vi "Set Variant.vi"(8 "error in (no error)":errorcluster, 10 "Variant":variant, 11 "int32 in":refnum<class "int32.lvclass">) -> (0 "error out":errorcluster, 3 "int32 out":refnum<class "int32.lvclass">)   [LabVIEW 2020, in "Protobuf RAW.lvlib" / "int32.lvclass"]
uses:
  int32.lvclass
  int32.lvclass/int32.ctl
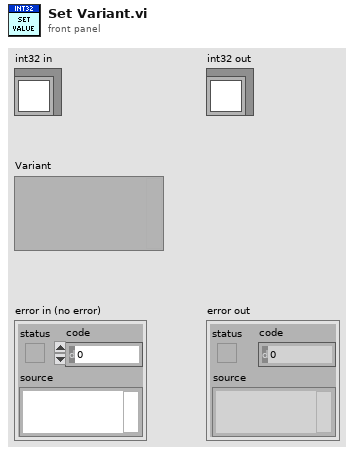
[diagram p1: front panel]
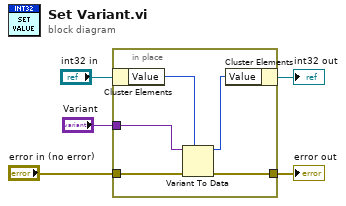
[diagram p0: block diagram]
diagram:
  n1 = in-place {
    in-place-border: "error in (no error)" -> [w10]
    in-place-border: [w9] -> w2
    in-place-border: "Variant" -> [w8]
    n2 = in-place-cluster #1("int32 in") -> ("Value"=w7:i32)
    n3 = Variant To Data(error in=w10, type=w7, Variant=w8) -> (data=w6:i32, error out=w9:errorcluster)
    n4 = in-place-cluster #1("Value"=w6) -> (→"int32 out":refnum<class "int32.lvclass">)
  }
  "error out" <- w2
